vi "RetrunClassReference.vi"(8 "error in (no error)":errorcluster, 11 "CreateClass in":refnum<class "CreateClass.lvclass">) -> (0 "error out":errorcluster, 2 "ClassRef":refnum<vi>, 3 "CreateClass out":refnum<class "CreateClass.lvclass">)   [LabVIEW 2020, in "Mermaid.lvlib" / "CreateClass.lvclass"]
uses:
  CreateClass.lvclass
  CreateClass.lvclass/CreateClass.ctl
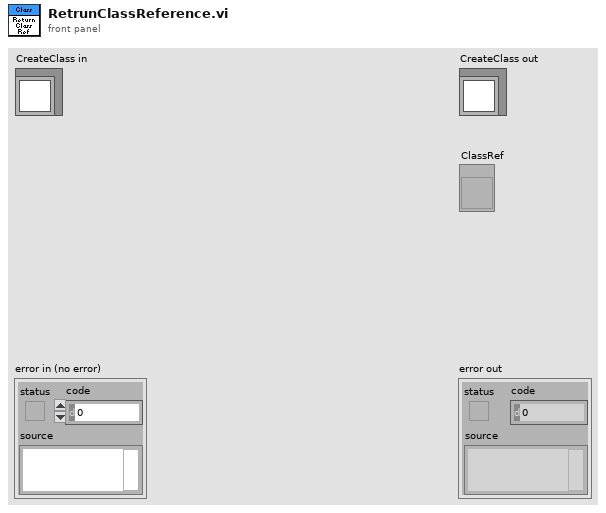
[diagram p1: front panel]
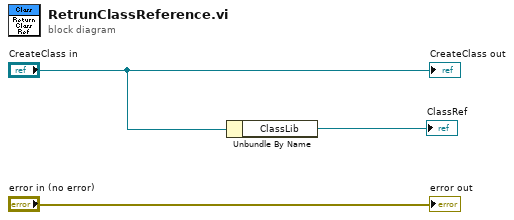
[diagram p0: block diagram]
diagram:
  n1 = Unbundle By Name("CreateClass in") -> ("ClassLib"=→"ClassRef":refnum<vi>)
  "error out" <- "error in (no error)"
  "CreateClass out" <- "CreateClass in"
